vi "Send Configure Resume Trigger [RT].vi"(6 "Trigger Slope (Positive)":i32(ring) caption="trigger slope (Positive)" items=["Positive", "Negative", "Either"], 7 "Message Priority (Normal)":T1=enum."Normal", 8 "error in (no error)":errorcluster, 9 "Trigger Source (None)":string(combo) caption="trigger source (None)", 10 "Channel Name (\"\")":string="CHANNEL1" caption="channel name (\"CHANNEL1\")", 11 "Message Enqueuer":refnum<class "Message Enqueuer.lvclass">) -> (0 "error out":errorcluster, 3 "Message Enqueuer out":refnum<class "Message Enqueuer.lvclass">)   [LabVIEW 2015, in "CS++Fgen.lvlib" / "Configure Resume Trigger [RT] Msg.lvclass"]
doc: "Sends the <B>CS++Fgen.lvlib:Configure Resume Trigger [RT] Msg.lvclass</B> message.\n\n<B>CS++Fgen.lvlib:CS++Fgen.lvclass:Configure Resume Trigger [RT].vi</B> Description:\n\nThis VI configures the properties that control the function generator's resume trigger. These properties are the resume trigger source and slope.\n\nA resume trigger resumes generation after it has been paused by a hold trigger, starting with the next point.\n\nNote:\n\n(1) This VI is part of the IviFgenResumeTrigger [RT] extension group."
uses:
  Configure Resume Trigger [RT] Msg.lvclass
  <vilib>/ActorFramework/Message Enqueuer/Message Enqueuer.lvclass
  <vilib>/ActorFramework/Message Enqueuer/Message Priority.ctl
  Configure Resume Trigger [RT] Msg.lvclass/Configure Resume Trigger [RT] Msg.ctl
  <vilib>/ActorFramework/Message Enqueuer/Message Enqueuer.lvclass/Message Enqueuer.ctl
  <vilib>/ActorFramework/Message Priority Queue/Priority Enqueue.vi
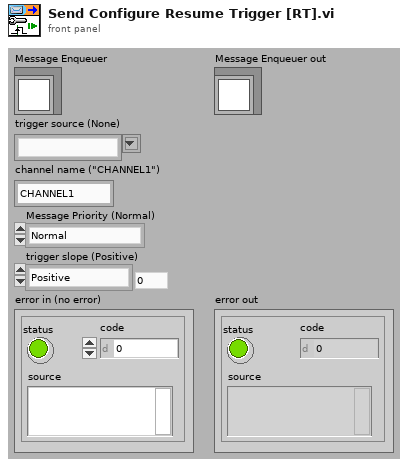
[diagram p1: front panel]
types:
  T1 = typedef "Actor Framework.lvlib/Message Enqueuer.lvclass/Message Priority.ctl" = enum16{"Low", "Normal", "High"}
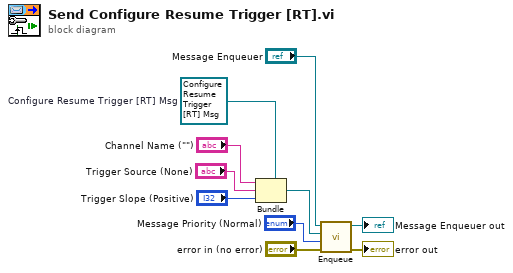
[diagram p0: block diagram]
diagram:
  w4 = refnum<class "Configure Resume Trigger [RT] Msg.lvclass"> refnum  # Configure Resume Trigger [RT] Msg
  n1 = Bundle(cluster=w4, "Channel Name (\"\")", "Trigger Source (None)", "Trigger Slope (Positive)") -> (w7:refnum<class "Configure Resume Trigger [RT] Msg.lvclass">)
  n2 = call <vilib>:"Enqueue.vi"("error in (no error)"="error in (no error)", "Message Priority (Normal)"="Message Priority (Normal)", "Message"=w7, "Message Enqueuer in"="Message Enqueuer") -> ("error out"=→"error out":errorcluster, "Message Enqueuer out"=→"Message Enqueuer out":refnum<class "Message Enqueuer.lvclass">)  [unwired: 6 in]
